vi "Test1.vi"() -> ()   [LabVIEW 2013]
panel:
  out "Numeric 2":dbl
  in  "Numeric":dbl
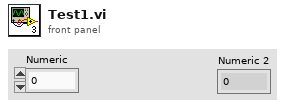
[diagram p1: front panel]
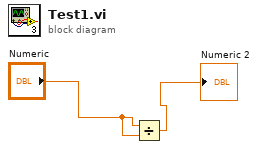
[diagram p0: block diagram]
diagram:
  n1 = Divide(x="Numeric", y="Numeric") -> (x/y=→"Numeric 2":dbl)
